vi "test-simpleTextodtFile.vi"() -> ()   [LabVIEW 2009]
uses:
  <vilib>/Utility/sysdir.llb/System Directory Type.ctl
  <vilib>/printing/ReportDocExtensions.llb/Append VI Block Diagram to Report (path).vi
  <vilib>/Utility/NIReport.llb/Append Report Text (str wrap).vi
  ooWriter/ooWriter.lvclass
  <vilib>/Utility/NIReport.llb/NI_report.lvclass
  <vilib>/Utility/NIReport.llb/NI_ReportGenerationCore.lvlib
panel:
  out "Writer error":errorcluster
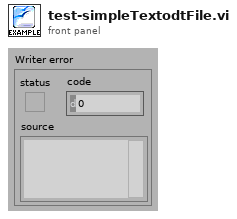
[diagram p1: front panel]
types:
  T1 = typedef "System Directory Type.ctl" = i32
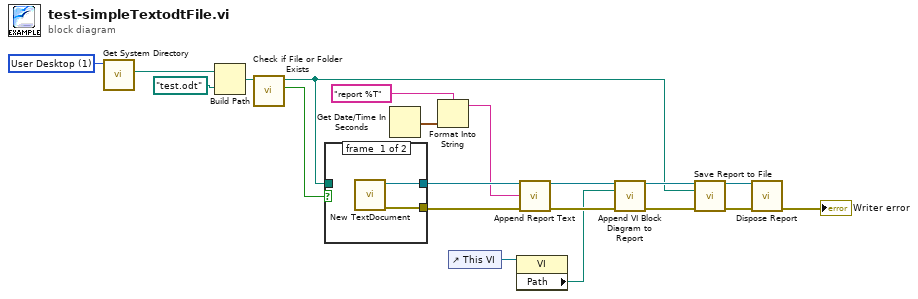
[diagram p0: block diagram]
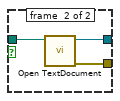
[diagram p2: hidden frame]
diagram:
  w11 = T1 1 items=["User Home", "User Desktop", "User Documents", "User Application Data", "User Preferences", "User Temporary", "Public Documents", "Public Application Data", "Public Preferences", "System Core Libraries", "System Installed Libraries", "Application Files", "Boot Volume Root"] ("system directory type")
  n1 = call <vilib>:"Get System Directory.vi"("system directory type"=w11) -> ("system directory"=w10:path)  [unwired: 10 in]
  n2 = Build Path(base path=w10, name or relative path=path "test.odt") -> (appended path=w8:path)
  n3 = call <vilib>:"Check if File or Folder Exists.vi"("path"=w8) -> ("file or folder exists?"=w7:bool, "dup path"=w4:path)  [unwired: 8 in, 1 out]
  n4 = case shown="True" w7 {
    tunnel: [w22 w24] -> w6
    tunnel: [w21 w23] -> w5
    tunnel: w4 -> [_ w25]
    frame #0 {
      n5 = call "New TextDocument.vi"() -> ("error out"=w21:errorcluster, "ooWriter out"=w22:refnum<class "ooWriter.lvclass">)  [unwired: 10 in]
    }
    frame #1 {
      n6 = call "Open TextDocument.vi"("filepath"=w25) -> ("error out"=w23:errorcluster, "ooWriter out"=w24:refnum<class "ooWriter.lvclass">)  [unwired: 9 in]
    }
  }
  n7 = Get Date/Time In Seconds() -> (seconds since 1Jan1904=w3:timestamp)
  n8 = Format Into String(format string="report %T" ("text"), w3) -> (resulting string=w1:string)  [unwired: 2 in, 1 out]
  n9 = control-ref of="This VI"() -> (w17:refnum<vi>)
  n10 = property class="VI"(reference=w17) -> ("Path"=w16:path)  [unwired: 1 in, 2 out]
  n11 = call-poly <vilib>:"Append Report Text.vi"("report in"=w6, "text"=w1, "error in (no error)"=w5) -> ("report out"=w20:refnum<class "ooWriter.lvclass">, "error out"=w18:errorcluster)  [unwired: 9 in, 2 out]
  n12 = call-poly <vilib>:"Append VI Block Diagram to Report.vi"("report in"=w20, "VI"=w16, "error in (no error)"=w18) -> ("report out"=w19:refnum<class "ooWriter.lvclass">, "error out"=w15:errorcluster)  [unwired: 8 in, 3 out]
  n13 = call-dynamic "Save Report to File.vi"("report in"=w19, "report file path"=w4, "error in (no error)"=w15) -> ("report out"=w14:refnum<class "ooWriter.lvclass">, "error out"=w13:errorcluster)  [unwired: 11 in]
  n14 = call-dynamic "Dispose Report.vi"("report in"=w14, "error in (no error)"=w13) -> ("error out"=→"Writer error":errorcluster)  [unwired: 13 in]
